vi "Store New Running Measurement.vi"(8 "error in (no error)":errorcluster, 9 "Caller-To-Actor Enqueuer":refnum<class "Message Enqueuer.lvclass">, 10 "name":string, 11 "Mag Lab Measure Controller in":refnum<class "Mag Lab Measure Controller.lvclass">) -> (0 "error out":errorcluster, 3 "Mag Lab Measure Controller out":refnum<class "Mag Lab Measure Controller.lvclass">)   [LabVIEW 2015, in "Mag Lab Measure Controller.lvclass"]
uses:
  Mag Lab Measure Controller.lvclass
  <vilib>/ActorFramework/Message Enqueuer/Message Enqueuer.lvclass
  Mag Lab Measure Controller.lvclass/Mag Lab Measure Controller.ctl
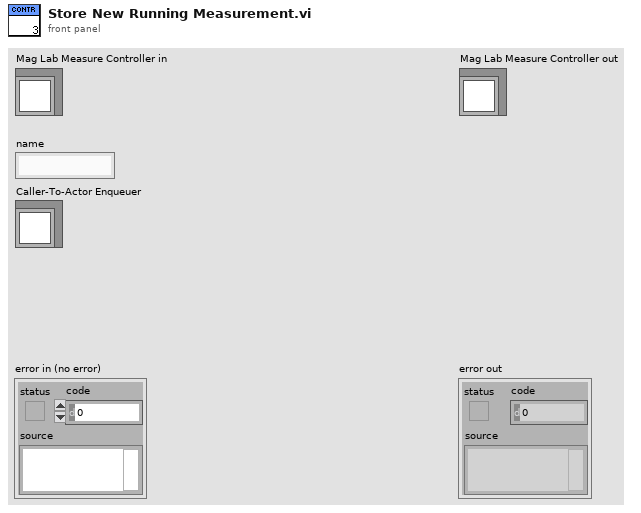
[diagram p1: front panel]
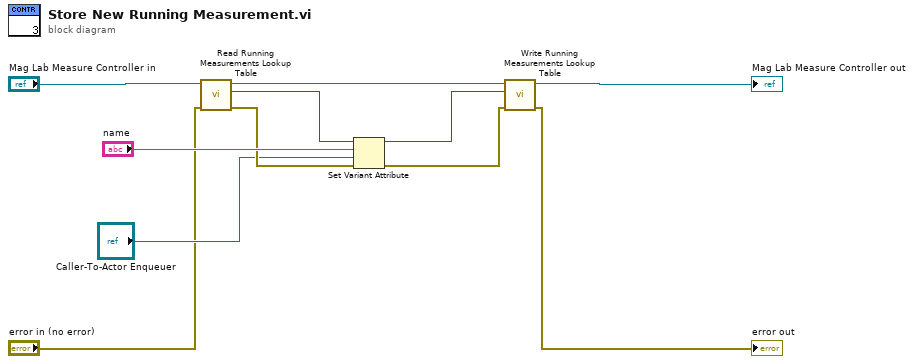
[diagram p0: block diagram]
diagram:
  n1 = call "Read Running Measurements Lookup Table.vi"("error in (no error)"="error in (no error)", "Mag Lab Measure Controller in"="Mag Lab Measure Controller in") -> ("error out"=w7:errorcluster, "Running Measurements Queue Lookup Table"=w8:variant, "Mag Lab Measure Controller out"=w11:refnum<class "Mag Lab Measure Controller.lvclass">)  [unwired: 7 in]
  n2 = Set Variant Attribute(Variant=w8, name="name", value="Caller-To-Actor Enqueuer", error in=w7) -> (Variant out=w10:variant, error out=w6:errorcluster)  [unwired: 1 out]
  n3 = call "Write Running Measurements Lookup Table.vi"("error in (no error)"=w6, "Running Measurements Queue Lookup Table"=w10, "Mag Lab Measure Controller in"=w11) -> ("error out"=→"error out":errorcluster, "Mag Lab Measure Controller out"=→"Mag Lab Measure Controller out":refnum<class "Mag Lab Measure Controller.lvclass">)  [unwired: 7 in]
